vi "SpecAn Span Set.vi"(0 "VISA In":refnum<visa-resource-name>, 5 "Error In":errorcluster, 6 "Span (Hz)":dbl=100000000.0 format="%#_6p") -> (14 "VISA Out":refnum<visa-resource-name>, 19 "Error Out":errorcluster)   [LabVIEW 2015]
uses:
  Controls/FGV Action SpecAn Model.ctl
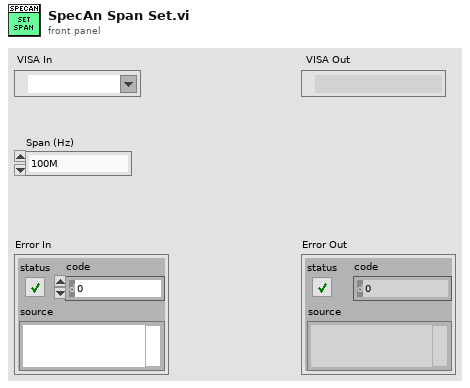
[diagram p1: front panel]
types:
  T1 = typedef "FGV Action SpecAn Model.ctl" = enum16{"Get", "Set"}
  T2 = typedef "SpecAn Model.ctl" = enum16{"E4440", "N9030"}
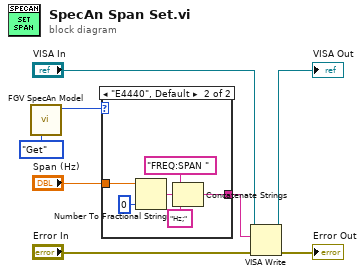
[diagram p0: block diagram]
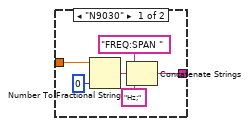
[diagram p2: hidden frame]
diagram:
  n1 = call "FGV SpecAn Model.vi"("Action"=FGV_Action_SpecAn_Model."Get") -> ("SA Model"=w1:T2)  [unwired: 6 in, 1 out]
  n2 = case shown="\"E4440\", Default" w1 {
    tunnel: "Span (Hz)" -> [w14 w20]
    tunnel: [w9 w15] -> w3
    frame "N9030" {
      n3 = Number To Fractional String(number=w14, precision (6)=i16 0) -> (F-format string=w10:string)  [unwired: 2 in]
      n4 = Concatenate Strings("FREQ:SPAN " ("format string"), w10, "Hz;" ("format string")) -> (w9:string)
    }
    frame "E4440", Default {
      n5 = Number To Fractional String(number=w20, precision (6)=i16 0) -> (F-format string=w16:string)  [unwired: 2 in]
      n6 = Concatenate Strings("FREQ:SPAN " ("format string"), w16, "Hz;" ("format string")) -> (w15:string)
    }
  }
  n7 = VISA Write(VISA resource name="VISA In", write buffer=w3, error in (no error)="Error In") -> (VISA resource name out=→"VISA Out":refnum<visa-resource-name>, error out=→"Error Out":errorcluster)  [unwired: 1 out]
